vi "Drop Through Click.vi"(8 "error in (no error)":errorcluster, 11 "hwnd":u32) -> (0 "error out":errorcluster)   [LabVIEW 2016, in "LV MDI.lvclass"]
uses:
  LV MDI.lvclass
  user32.dll
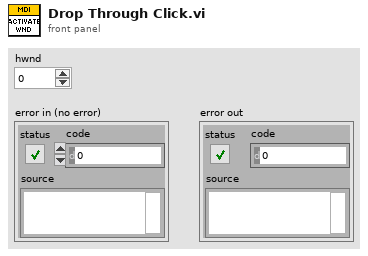
[diagram p1: front panel]
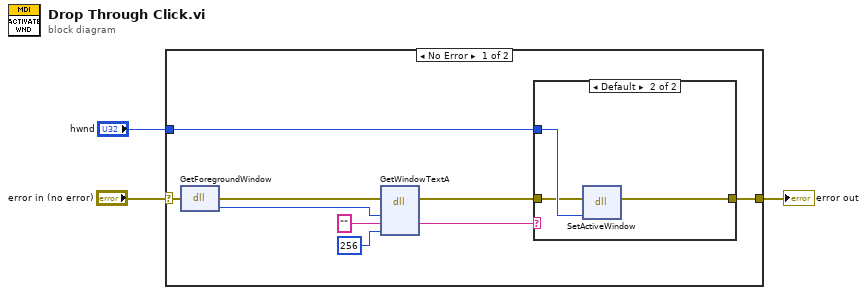
[diagram p0: block diagram]
diagram:
  n1 = case shown="No Error" "error in (no error)" {
    selector: "error in (no error)" -> [w10 w17]
    tunnel: [w5 w17] -> w2
    tunnel: "hwnd" -> [w4 _]
    frame No Error {
      n2 = dll-call lib="user32.dll" fn="GetForegroundWindow"(error in=w10) -> (error out=w9:errorcluster, "hwnd"=w8:u32)  [unwired: 2 in, 1 out]
      n3 = dll-call lib="user32.dll" fn="GetWindowTextA"(error in=w9, "hwnd"=w8, "lpString"="", "nMaxcount"=256) -> (error out=w11:errorcluster, "lpString"=w12:string)  [unwired: 5 in, 1 out]
      n4 = case shown="Default" w12 {
        tunnel: w4 -> [_ w16]
        tunnel: [w13 w15] -> w5
        tunnel: w11 -> [w13 w14]
        frame "Open" {
        }
        frame Default {
          n5 = dll-call lib="user32.dll" fn="SetActiveWindow"(error in=w14, "hwnd"=w16) -> (error out=w15:errorcluster)  [unwired: 4 in, 1 out]
        }
      }
    }
    frame Error {
    }
  }
  "error out" <- w2
